vi "Sample Timer Functions.vi"(8 "Next Time In":dbl format="%.1f", 9 "Start Time":dbl format="%.1f", 10 "DAQ Units":u16(ring) items=["Mins", "Hrs"], 11 "DAQ Period":u32) -> (0 "Next Time Out":dbl format="%.1f", 1 "New Time Out":dbl format="%.1f", 2 "Sample Now":bool, 3 "Elapsed Hours":dbl format="%.1f", 4 "DAQ Period (secs)":dbl, 5 "Time":timestamp=timestamp(3199635000.25 s since 1904-01-01) format="%<%H:%M>T")   [LabVIEW 2013]
doc: "Computes values used for sample timing as follows:\n\nINPUTS\n DAQ Units - code for period units; 0=minutes, 1 = hours\n DAQ Period - the value in \"DAQ Units\" that the cell is sampled\n Start Time - the time in 1904 seconds the test was started\n Next Time In - the time in 1904 seconds when the next sample is scheduled\n\nOUTPUTS\n DAQ Period (secs) - the sampling periods in seconds\n Elapsed Hours - the elapsed hours since the test was started\n Sample Now - is TRUE if Next Time In is less than the current time, and FALSE otherwise\n Next Time Out - is the maximum of the Next Time In or the current time in 1904 seconds\n New Time Out - if Sample Now is TRUE, it is equal to either the current time plus the DAQ\n Period or the Next Time In plus the DAQ Period, whichever is greater.\n If Sample Now is FALSE, it is equal to either the Next Time In or the current\n time whichever is greater.\n Time - the clock time in 24-hour format; if Sample Now is TRUE, it is equal to the current time;\n if Sample Now is FALSE, it is the Next Time In minus the DAQ Period (last sample)."
panel:
  out "GreaterThan":bool
  out "Cur1904Secs":dbl format="%.1f"
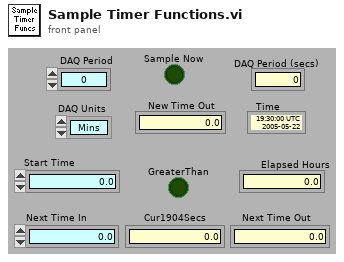
[diagram p1: front panel]
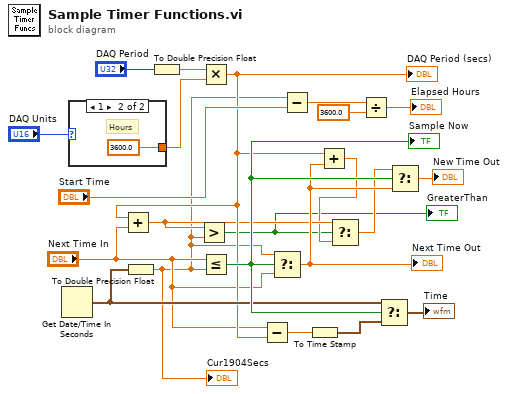
[diagram p0: block diagram]
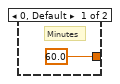
[diagram p2: hidden frame]
diagram:
  n1 = Get Date/Time In Seconds() -> (seconds since 1Jan1904=w11:timestamp)
  n2 = case shown="1" "DAQ Units" {
    tunnel: [60.0 3600.0] -> w19
    frame 0, Default {
      # "Minutes"
    }
    frame 1 {
      # "Hours"
    }
  }
  n3 = To Double Precision Float(number=w11) -> (double precision float=w3:dbl)
  "Cur1904Secs" <- w3
  n4 = To Double Precision Float(number="DAQ Period") -> (double precision float=w20:dbl)
  n5 = Multiply(x=w20, y=w19) -> (x*y=w10:dbl)
  "DAQ Period (secs)" <- w10
  n6 = Add(x=w10, y="Next Time In") -> (x+y=w7:dbl)
  n7 = Greater?(x=w7, y=w3) -> (0:w4:bool)
  "GreaterThan" <- w4
  n8 = Less Or Equal?(x="Next Time In", y=w3) -> (x <= y?=w13:bool)
  "Sample Now" <- w13
  n9 = Subtract(x="Next Time In", y=w10) -> (x-y=w2:dbl)
  n10 = Select(t=w3, s=w13, f="Next Time In") -> (s? t:f=w8:dbl)
  "Next Time Out" <- w8
  n11 = Subtract(x=w3, y="Start Time") -> (x-y=w17:dbl)
  n12 = To Time Stamp(1:w2) -> (0:w1:timestamp)
  n13 = Add(x=w10, y=w8) -> (x+y=w6:dbl)
  n14 = Select(t=w7, s=w4, f=w6) -> (s? t:f=w5:dbl)
  n15 = Divide(x=w17, y=3600.0) -> (x/y=→"Elapsed Hours":dbl)
  n16 = Select(t=w11, s=w13, f=w1) -> (s? t:f=→"Time":timestamp)
  n17 = Select(t=w5, s=w13, f=w8) -> (s? t:f=→"New Time Out":dbl)
